vi "Empty_bottle.vi"(0 "Odour bottles in":T1(array[cluster])) -> (7 "Odour bottles out":T1(array[cluster]))   [LabVIEW 2016]
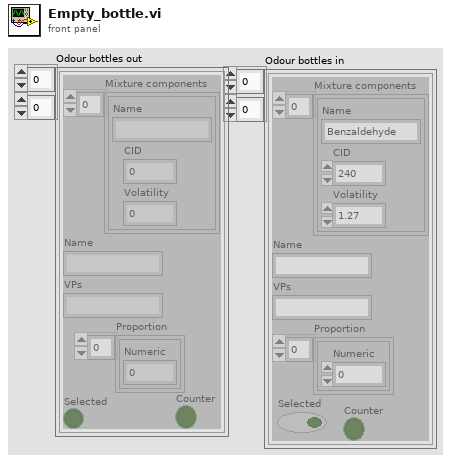
[diagram p1: front panel]
types:
  T1 = cluster{"Mixture components":cluster{"Name":string, "CID":i32, "Volatility":dbl}[], "Name":string, "VPs":string, "Proportion":cluster{"Numeric":dbl}[], "Selected":bool, "Counter":bool}[][]
  T2 = cluster{"Name":string, "CID":i32, "Volatility":dbl}[]
  T3 = cluster{"Mixture components":cluster{"Name":string, "CID":i32, "Volatility":dbl}[], "Name":string, "VPs":string, "Proportion":cluster{"Numeric":dbl}[], "Selected":bool, "Counter":bool}
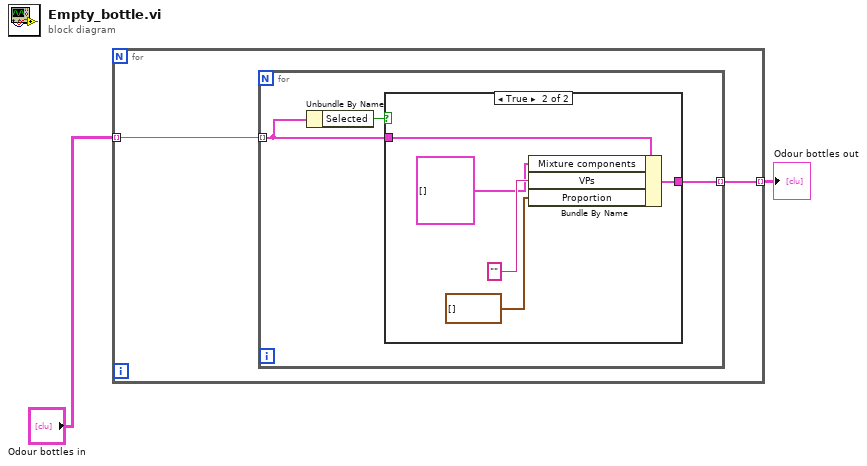
[diagram p0: block diagram]
diagram:
  n1 = for {
    tunnel: "Odour bottles in" -> [w4] mode=indexing
    tunnel: [w3] -> w1 mode=indexing
    n2 = for {
      tunnel: w4 -> [w7] mode=indexing
      tunnel: [w5] -> w3 mode=indexing
      n3 = Unbundle By Name(w7) -> ("Selected"=w6:bool)
      n4 = case shown="True" w6 {
        tunnel: w7 -> [w8 w13]
        tunnel: [w8 w10] -> w5
        frame False {
        }
        frame True {
          n5 = Bundle By Name(cluster=w13, "Mixture components"=T2 [], "VPs"="", "Proportion"=cluster{"Numeric":dbl}[] []) -> (w10:T3)
        }
      }
    }
  }
  "Odour bottles out" <- w1
